vi "test Get All Parameters.vi"(8 "error in":errorcluster, 11 "TestCase in":refnum<class "Scripting.lvclass">) -> (0 "error out":errorcluster, 3 "TestCase out":refnum<class "Scripting.lvclass">)   [LabVIEW 2020, in "Scripting.lvclass"]
uses:
  Scripting.lvclass
  Scripting.lvclass/Scripting.ctl
  <vilib>/addons/_JKI Toolkits/VI Tester/TestCase.llb/TestCase.lvclass
  Scripting/Ballard ARINC 429 Scripting.lvlib
  C:/Program Files (x86)/National Instruments/LabVIEW 2020/vi.lib/addons/_JKI Toolkits/VI Tester/TestCase.llb/TestCase.lvclass
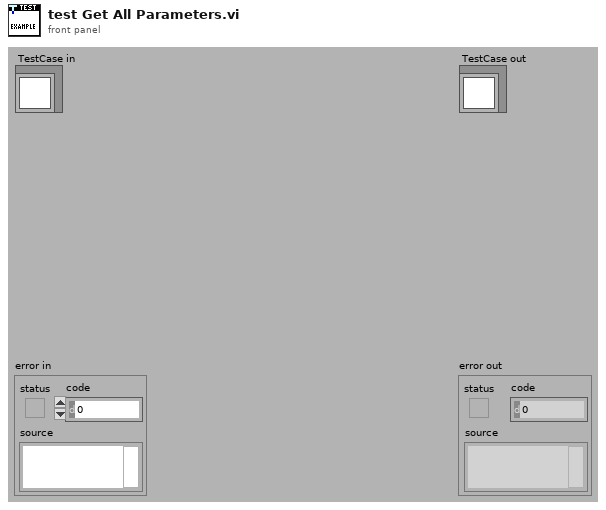
[diagram p1: front panel]
types:
  T1 = typedef "Custom Device API.lvlib/Custom Device Item Ref.ctl" = u64
  T2 = typedef "Parameter Definition.ctl" = cluster{"start index":i32, "size":i32, "encoding":T3, "signed":bool, "scale multiplier":dbl, "scale offset":dbl}
  T3 = typedef "Encoding and Decoding.lvlib/Encoding.ctl" = enum16{"BNR", "BCD", "Discrete"}
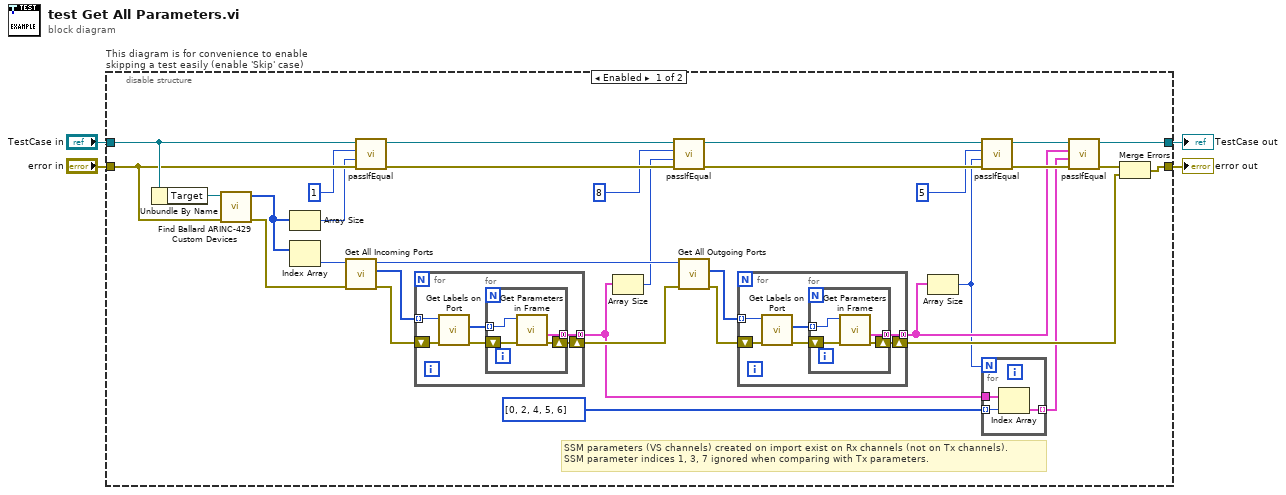
[diagram p0: block diagram]
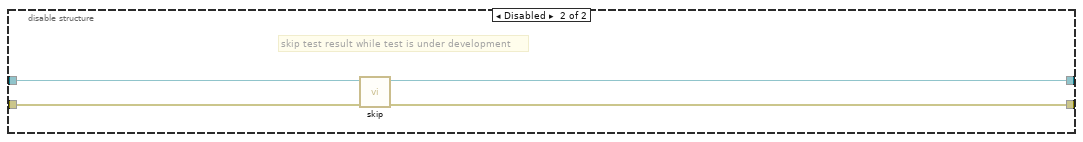
[diagram p2: hidden frame]
diagram:
  n1 = disable-structure "This diagram is for convenience to enable skipping a test easily (enable 'Skip' case)" shown="Enabled" {
    disable-tunnel: "TestCase in" -> [w34 w63]
    disable-tunnel: [w24 w61] -> w1
    disable-tunnel: [w25 w62] -> w3
    disable-tunnel: "error in" -> [w33 w60]
    frame Enabled {
      # "SSM parameters (VS channels) created on import exist on Rx channels (not on Tx channels).\nSSM parameter indices 1, 3, 7 ignored when comparing with Tx parameters."
      n2 = Unbundle By Name(w34) -> ("Target"=w36:refnum<k24>)
      n3 = call "Find Ballard ARINC-429 Custom Devices.vi"("error in"=w33, "target"=w36) -> ("error out"=w27:errorcluster, "Ballard ARINC-429 custom devices"=w32:u64[])  [unwired: 8 in]
      n4 = Array Size(array=w32) -> (size(s)=w30:i32)
      n5 = Index Array(array=w32) -> (element=w35:u64)  [unwired: 1 in]
      n6 = call "Get All Incoming Ports.vi"("error in"=w27, "Ballard ARINC 429 ref"=w35) -> ("error out"=w18:errorcluster, "Port refs"=w17:T1[], "Ballard ARINC 429 ref out"=w26:T1)  [unwired: 7 in]
      n7 = call-dynamic "passIfEqual.vi"("error in (no error)"=w33, "y"=w30, "x"=1 ("size(s)"), "TestCase in"=w34) -> ("error out"=w28:errorcluster, "TestCase out"=w29:refnum<class "Scripting.lvclass">)  [unwired: 6 in]
      n8 = for {
        tunnel: [w54] -> w7 mode=concatenating
        shift-right: [w55] -> w22
        shift-left: w18 -> [w53]
        tunnel: w17 -> [w50] mode=indexing
        n9 = call "Get Labels on Port.vi"("error in"=w53, "port ref"=w50) -> ("error out"=w52:errorcluster, "label references"=w51:T1[])  [unwired: 6 in, 2 out]
        n10 = for {
          tunnel: [w58] -> w54 mode=concatenating
          shift-right: [w59] -> w55
          shift-left: w52 -> [w57]
          tunnel: w51 -> [w56] mode=indexing
          n11 = call "Get Parameters in Frame.vi"("error in"=w57, "frame ref in"=w56) -> ("error out"=w59:errorcluster, "parameter definitions"=w58:T2[])  [unwired: 6 in, 2 out]
        }
      }
      n12 = Array Size(array=w7) -> (size(s)=w11:i32)
      n13 = call-dynamic "passIfEqual.vi"("error in (no error)"=w28, "y"=w11, "x"=8 ("size(s)"), "TestCase in"=w29) -> ("error out"=w19:errorcluster, "TestCase out"=w20:refnum<class "Scripting.lvclass">)  [unwired: 6 in]
      n14 = call "Get All Outgoing Ports.vi"("error in"=w22, "Ballard ARINC 429 ref"=w26) -> ("error out"=w13:errorcluster, "Port refs"=w14:T1[])  [unwired: 7 in, 1 out]
      n15 = for {
        tunnel: [w44] -> w9 mode=concatenating
        shift-right: [w45] -> w12
        shift-left: w13 -> [w43]
        tunnel: w14 -> [w40] mode=indexing
        n16 = call "Get Labels on Port.vi"("error in"=w43, "port ref"=w40) -> ("error out"=w42:errorcluster, "label references"=w41:T1[])  [unwired: 6 in, 2 out]
        n17 = for {
          tunnel: [w48] -> w44 mode=concatenating
          shift-right: [w49] -> w45
          shift-left: w42 -> [w47]
          tunnel: w41 -> [w46] mode=indexing
          n18 = call "Get Parameters in Frame.vi"("error in"=w47, "frame ref in"=w46) -> ("error out"=w49:errorcluster, "parameter definitions"=w48:T2[])  [unwired: 6 in, 2 out]
        }
      }
      n19 = Array Size(array=w9) -> (size(s)=w8:i32)
      n20 = call-dynamic "passIfEqual.vi"("error in (no error)"=w19, "y"=w8, "x"=5 ("size(s)"), "TestCase in"=w20) -> ("error out"=w15:errorcluster, "TestCase out"=w16:refnum<class "Scripting.lvclass">)  [unwired: 6 in]
      n21 = for {
        N: w8 -> [_]
        tunnel: w7 -> [w39]
        tunnel: i32[] [0, 2, 4, 5, 6] -> [w38] mode=indexing
        tunnel: [w37] -> w5 mode=indexing
        n22 = Index Array(array=w39, index=w38) -> (element=w37:T2)
      }
      n23 = call-dynamic "passIfEqual.vi"("error in (no error)"=w15, "y"=w5, "x"=w9, "TestCase in"=w16) -> ("error out"=w23:errorcluster, "TestCase out"=w24:refnum<class "Scripting.lvclass">)  [unwired: 6 in]
      n24 = Merge Errors(w23, w12) -> (w25:errorcluster)
    }
    frame Disabled {
      # "skip test result while test is under development"
      n25 = call <vilib>:"skip.vi"("error in (no error)"=w60, "TestCase in"=w63) -> ("error out"=w62:errorcluster, "TestCase out"=w61:refnum<class "Scripting.lvclass">)  [unwired: 8 in]
    }
  }
  "error out" <- w3
  "TestCase out" <- w1
